vi "Get Buffer Configuration.vi"(10 "Encoder Data Description":string, 11 "Buffer Configuration in":T1) -> (2 "Type":T3, 3 "Buffer Configuration out":T1)   [LabVIEW 2021, in "CIF_CIPC_Chn.lvclass"]
uses:
  CIF_CIPC_Chn.lvclass
  <vilib>/Utility/Data Type/Type Definitions/Data Type.ctl
  <vilib>/Utility/error.llb/Trim Whitespace.vi
  CIF_CIPC_Chn.lvclass/CIF_CIPC_Chn.ctl
  <vilib>/CIF Foundation/CIF CIPC/CIF_NI_CIPC.lvlib
  <vilib>/Utility/Data Type/NI_Data Type.lvlib
  Typedef/Buffer Configuration Data.ctl
  <vilib>/CIF Foundation/CIF CIPC/TypeDefs/Backpressure References.ctl
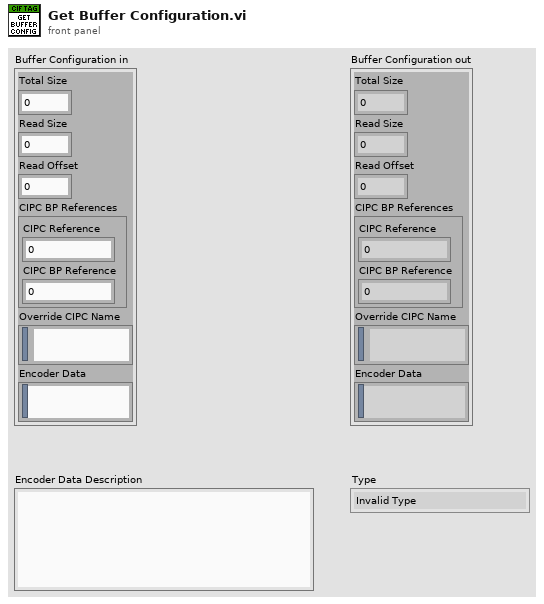
[diagram p1: front panel]
types:
  T1 = typedef "CIF_CIPC_Chn.lvclass/Buffer Configuration Data.ctl" = cluster{"Total Size":u32, "Read Size":u32, "Read Offset":u32, "CIPC BP References":T2, "Override CIPC Name":string, "Encoder Data":string}
  T2 = typedef "CIF_NI_CIPC.lvlib/Backpressure References.ctl" = cluster{"CIPC Reference":u64, "CIPC BP Reference":u64}
  T3 = typedef "NI_Data Type.lvlib/Data Type.ctl" = enum8{"Invalid Type", "Void", "I8", "I16", "I32", "I64", "U8", "U16", "U32", "U64", "Single Float", "Double Float", "Extended Float", "Single Complex", "Double Complex", "Extended Complex", "Enum U8", "Enum U16", "Enum U32", "Enum U64", "Single Float With Unit", "Double Float With Unit", "Extended Float With Unit", "Single Complex with Unit", "Double Complex with Unit", "Extended Complex with Unit", "Boolean", "String", "Path", "Picture", "Tag", "Array", "Cluster", "Variant", "LV Variant", "Waveform", "Timestamp", "Digital Waveform", "Digital Data", "ExpressData", "Refnum", "External Data", "VI", "Poly VI", "LabVIEW Class Instance", "Fixed Point", "Set Collection", "Map Collection"}
  T4 = typedef "CIF_NI_CIPC.lvlib/Data Element.ctl" = cluster{"Name":string, "Type":T3, "Size":u32, "Offset":u32}
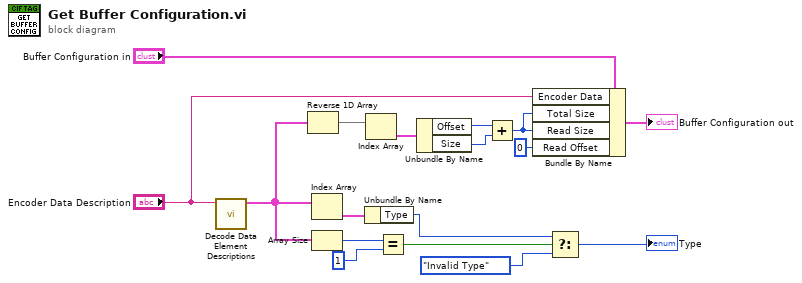
[diagram p0: block diagram]
diagram:
  n1 = call <vilib>:"Decode Data Element Descriptions.vi"("Encoder Data Description"="Encoder Data Description") -> ("Data Elements"=w14:T4[])  [unwired: 10 in]
  n2 = Reverse 1D Array(array=w14) -> (reversed array=w13:T4[])
  n3 = Index Array(array=w14) -> (element=w15:T4)  [unwired: 1 in]
  n4 = Array Size(array=w14) -> (size(s)=w17:i32)
  n5 = Unbundle By Name(w15) -> ("Type"=w5:T3)
  n6 = Index Array(array=w13) -> (element=w12:T4)  [unwired: 1 in]
  n7 = Equal?(x=w17, y=1) -> (x = y?=w4:bool)
  n8 = Unbundle By Name(w12) -> ("Offset"=w11:u32, "Size"=w10:u32)
  n9 = Add(x=w11, y=w10) -> (x+y=w8:u32)
  n10 = Bundle By Name(cluster="Buffer Configuration in", "Encoder Data"="Encoder Data Description", "Total Size"=w8, "Read Size"=w8, "Read Offset"=u32 0) -> (→"Buffer Configuration out":T1)
  n11 = Select(t=w5, s=w4, f=Data_Type."Invalid Type") -> (s? t:f=→"Type":T3)
